vi "shiyan.vi"() -> ()   [LabVIEW 2013]
uses:
  <vilib>/gmath/NI_Gmath.lvlib
panel:
  out "Y":dbl
  in  "X":dbl
  out "XY图":cluster{i32[], dbl[]}(graph)
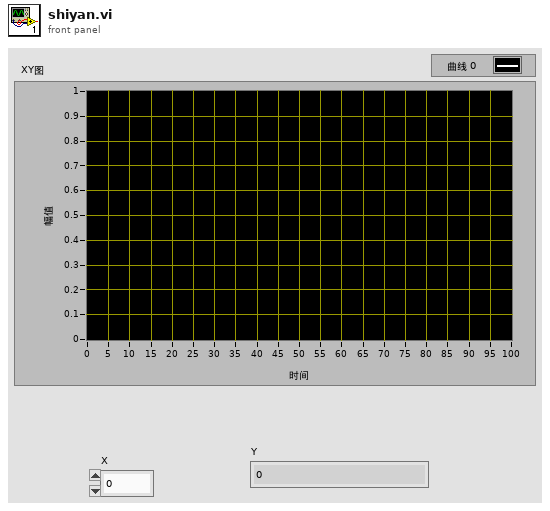
[diagram p1: front panel]
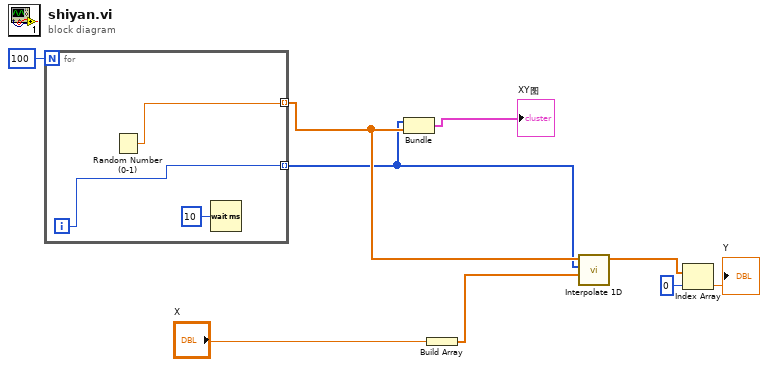
[diagram p0: block diagram]
diagram:
  n1 = for {
    N: 100 -> [_]
    tunnel: [w12] -> w7 mode=indexing
    tunnel: [w10] -> w6 mode=indexing
    i -> [w10]
    n2 = Random Number (0-1)() -> (number: 0 to 1=w12:dbl)
    n3 = Wait (ms)(milliseconds to wait=u32 10 ("等待时间（毫秒）")) -> ()  [unwired: 1 out]
  }
  n4 = Bundle(w6, w7) -> (→"XY图":cluster{i32[], dbl[]})  [unwired: 1 in]
  n5 = Build Array("X") -> (w4:dbl[])
  n6 = call <vilib>:"Interpolate 1D.vi"("xi"=w4, "X"=w6, "Y"=w7) -> ("yi"=w3:dbl[])  [unwired: 6 in, 2 out]
  n7 = Index Array(array=w3, index=0 ("索引")) -> (element=→"Y":dbl)
